vi "QuadCombine (SubVI).vi"(0 "roi":dbl[](array[numeric]), 1 "# of radial bins":i32, 5 "radial bins/pixel":dbl, 7 "window":dbl[](array[numeric]), 11 "profiles":dbl[][](array[numeric]), 12 "pre-xy (pixels)":dbl[](array[numeric])) -> (3 "Position Correction":dbl[](array[numeric]), 6 "Position (pixels)":dbl[](array[numeric]), 10 "radial profile":dbl[](array[numeric]))   [LabVIEW 2011, in "OfflineTracker.lvlib"]
uses:
  OfflineTracker.lvlib
  <vilib>/Analysis/5stat.llb/RMS (DBL).vi
  <vilib>/Analysis/2dsp.llb/Real FFT.vi
  <vilib>/Analysis/2dsp.llb/Inverse Real FFT.vi
  <vilib>/Analysis/NI_AALPro.lvlib
panel:
  out "Waveform Graph 2":dbl[][](graph)
  out "Waveform Graph":dbl[][](graph)
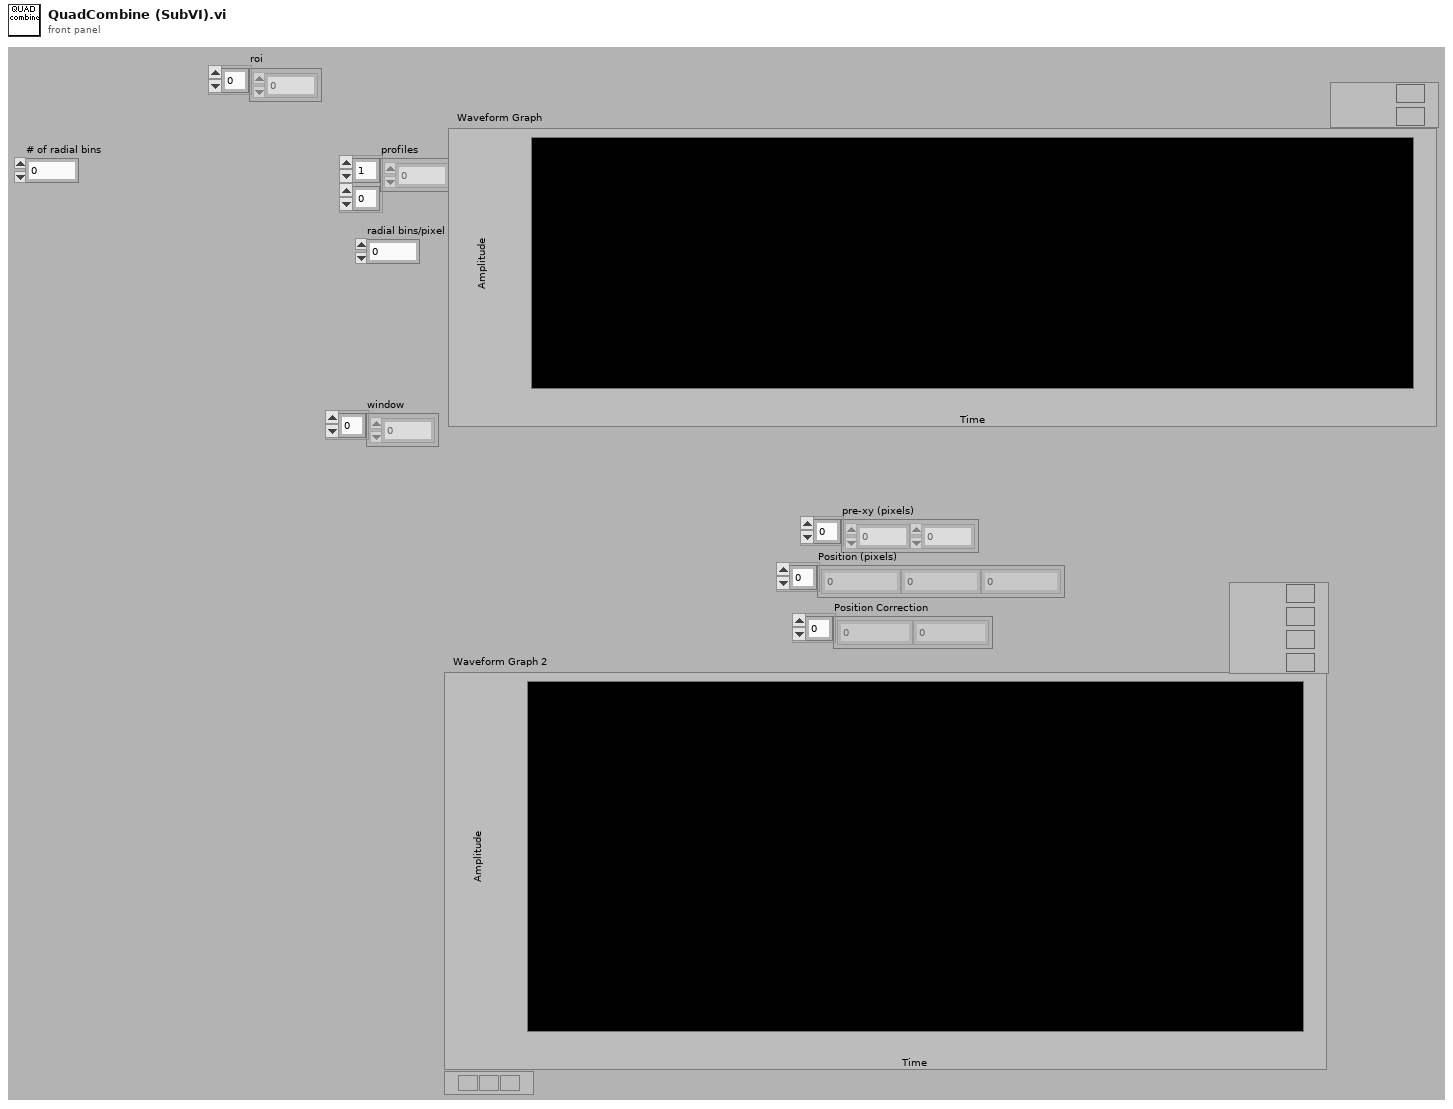
[diagram p1: front panel]
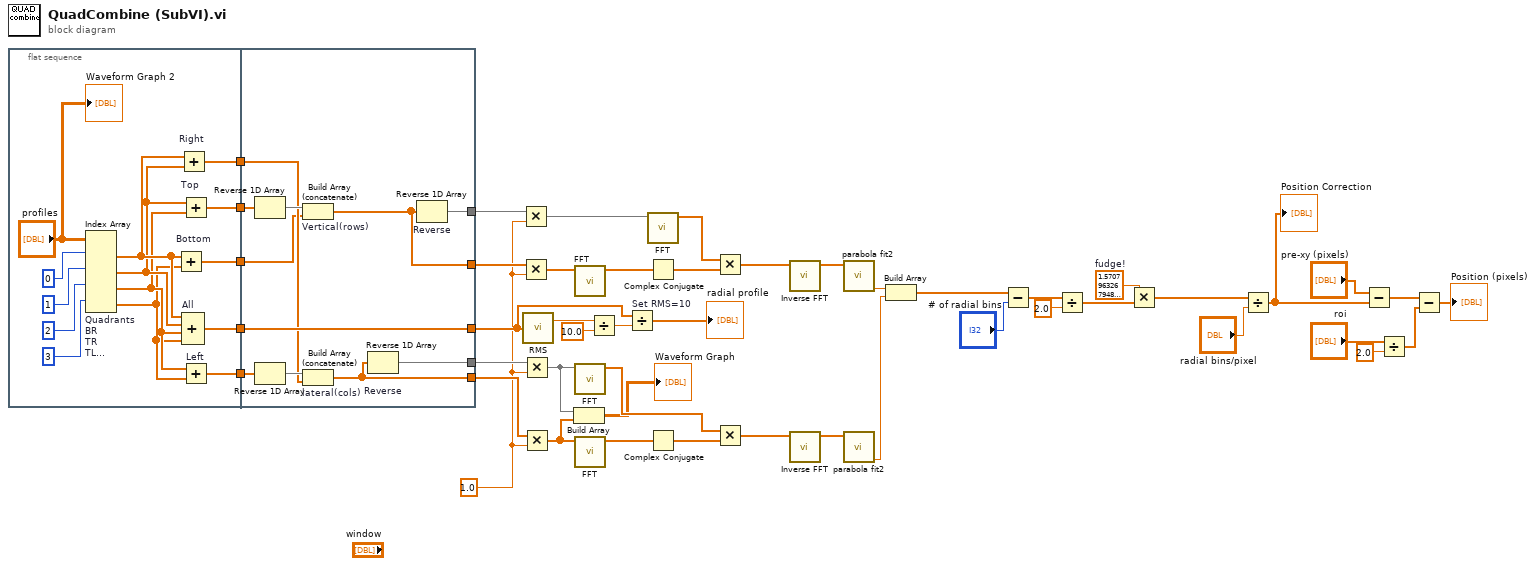
[diagram p0: block diagram]
diagram:
  w1 = 1.0 ("y")
  w11 = 1.5707963267948966  # fudge!
  n1 = flat-sequence {
    tunnel: [w50] -> w36
    tunnel: [w49] -> w35
    tunnel: [w56] -> w34
    tunnel: [w51] -> w30
    tunnel: [w48] -> w29
    tunnel: [w69] -> w9
    tunnel: [w67] -> w3
    tunnel: [w66] -> w5
    tunnel: [w68] -> w7
    tunnel: w36 -> [w63]
    tunnel: w35 -> [w72]
    tunnel: w34 -> [w65]
    tunnel: [w64] -> w32
    tunnel: w30 -> [w64]
    tunnel: w29 -> [w62]
    frame #0 {
      n2 = Index Array "Quadrants\nBR\nTR\nTL\nBL"(array="profiles", index (row) #1=0 ("index (row)"), index (row) #2=1 ("index (row)"), index (row) #3=2 ("disabled index (col)"), index (row) #4=3 ("index (row)")) -> (element #1=w55:dbl[], element #2=w54:dbl[], element #3=w53:dbl[], element #4=w52:dbl[])  [unwired: 4 in]
      n3 = Add "Bottom"(x=w55, y=w52) -> (x+y=w48:dbl[])
      n4 = Add "Right"(x=w55, y=w54) -> (x+y=w50:dbl[])
      n5 = Add "Top"(x=w54, y=w53) -> (x+y=w49:dbl[])
      n6 = Add "Left"(x=w53, y=w52) -> (x+y=w56:dbl[])
      n7 = Compound Arithmetic op=ADD "All"(w55, w54, w53, w52) -> (w51:dbl[])
      "Waveform Graph 2" <- "profiles"
    }
    frame #1 {
      n8 = Reverse 1D Array(array=w72) -> (reversed array=w71:dbl[])
      n9 = Reverse 1D Array(array=w65) -> (reversed array=w70:dbl[])
      n10 = Build Array (concatenate) "Vertical(rows)"(w71, w62) -> (w66:dbl[])
      n11 = Build Array (concatenate) "lateral(cols)"(w70, w63) -> (w69:dbl[])
      n12 = Reverse 1D Array "Reverse"(array=w69) -> (reversed array=w68:dbl[])
      n13 = Reverse 1D Array "Reverse"(array=w66) -> (reversed array=w67:dbl[])
    }
  }
  n14 = Multiply(x=w3, y=w1) -> (x*y=w2:dbl[])
  n15 = Multiply(x=w5, y=w1) -> (x*y=w4:dbl[])
  n16 = Multiply(x=w7, y=w1) -> (x*y=w6:dbl[])
  n17 = Multiply(x=w9, y=w1) -> (x*y=w8:dbl[])
  n18 = call-poly <vilib>:"RMS.vi"("X"=w32) -> ("rms value"=w39:dbl)  [unwired: 1 out]
  n19 = Build Array(w6, w8) -> (→"Waveform Graph":dbl[][])
  n20 = call-poly <vilib>:"FFT.vi"("X"=w4) -> ("FFT {X}"=w44:cdb[])  [unwired: 2 in, 8 out]
  n21 = call-poly <vilib>:"FFT.vi"("X"=w6) -> ("FFT {X}"=w42:cdb[])  [unwired: 2 in, 8 out]
  n22 = call-poly <vilib>:"FFT.vi"("X"=w8) -> ("FFT {X}"=w40:cdb[])  [unwired: 2 in, 8 out]
  n23 = Divide(x=w39, y=10.0) -> (x/y=w37:dbl)
  n24 = Divide "Set RMS=10"(x=w32, y=w37) -> (x/y=→"radial profile":dbl[])
  n25 = call-poly <vilib>:"FFT.vi"("X"=w2) -> ("FFT {X}"=w46:cdb[])  [unwired: 2 in, 8 out]
  n26 = Complex Conjugate(1:w44) -> (0:w45:cdb[])
  n27 = Complex Conjugate(1:w40) -> (0:w41:cdb[])
  n28 = Multiply(x=w46, y=w45) -> (x*y=w47:cdb[])
  n29 = Multiply(x=w42, y=w41) -> (x*y=w43:cdb[])
  n30 = call-poly <vilib>:"Inverse FFT.vi"("FFT {X}"=w47) -> ("X"=w26:dbl[])  [unwired: 1 in, 9 out]
  n31 = call-poly <vilib>:"Inverse FFT.vi"("FFT {X}"=w43) -> ("X"=w27:dbl[])  [unwired: 1 in, 9 out]
  n32 = call "parabola fit2.vi"("radial profile"=w26) -> ("Y focus"=w24:dbl)  [unwired: 7 out]
  n33 = call "parabola fit2.vi"("radial profile"=w27) -> ("Y focus"=w25:dbl)  [unwired: 7 out]
  n34 = Build Array(w24, w25) -> (w23:dbl[])
  n35 = Subtract(x=w23, y="# of radial bins") -> (x-y=w10:dbl[])
  n36 = Divide(x=w10, y=2.0) -> (x/y=w20:dbl[])
  n37 = Multiply(x=w11, y=w20) -> (x*y=w18:dbl[])
  n38 = Divide(x=w18, y="radial bins/pixel") -> (x/y=w19:dbl[])
  "Position Correction" <- w19
  n39 = Subtract(x="pre-xy (pixels)", y=w19) -> (x-y=w16:dbl[])
  n40 = Divide(x="roi", y=2.0 ("Y focus")) -> (x/y=w14:dbl[])
  n41 = Subtract(x=w16, y=w14) -> (x-y=→"Position (pixels)":dbl[])
